vi "功率电压图.vi"(11 "功率控制表":refnum<vi>) -> ()   [LabVIEW 2015]
panel:
  out "XY图":cluster{i32[], dbl[]}[](graph)
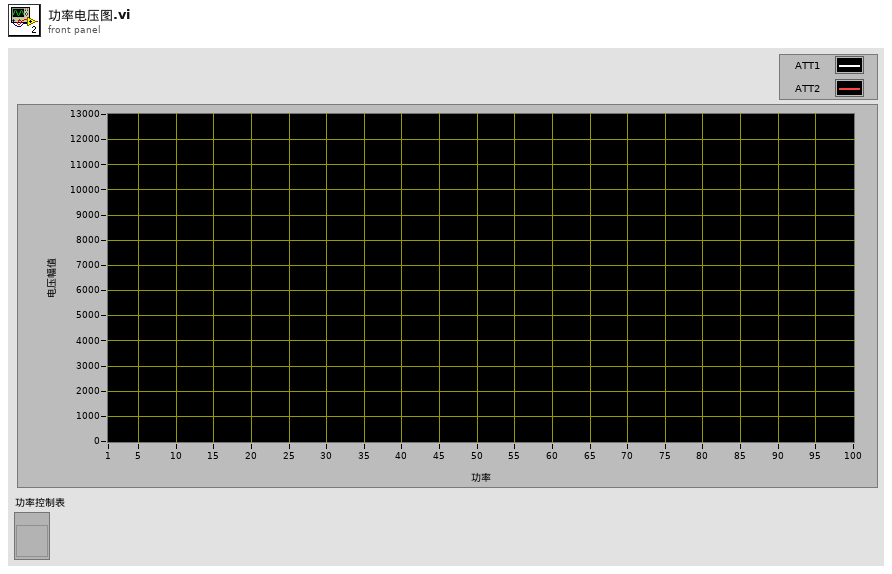
[diagram p1: front panel]
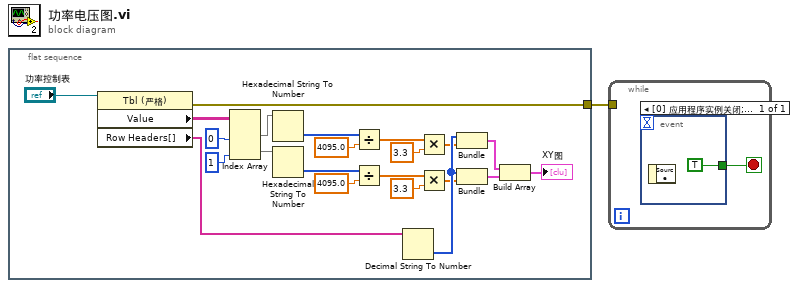
[diagram p0: block diagram]
diagram:
  n1 = flat-sequence {
    tunnel: [w12] -> w1
    frame #0 {
      n2 = property class="Tbl (严格)"(reference="功率控制表") -> (error out=w12:errorcluster, "Value"=w20:string[][], "Row Headers[]"=w21:string[])  [unwired: 1 in, 1 out]
      n3 = Index Array(array=w20, index (col) #1=0 ("禁用的索引 (列)"), index (col) #2=1 ("禁用的索引 (列)")) -> (element #1=w17:string[], element #2=w16:string[])  [unwired: 2 in]
      n4 = Hexadecimal String To Number(string=w17) -> (number=w8:u32[])  [unwired: 2 in, 1 out]
      n5 = Hexadecimal String To Number(string=w16) -> (number=w3:u32[])  [unwired: 2 in, 1 out]
      n6 = Divide(x=w8, y=4095.0) -> (x/y=w10:dbl[])
      n7 = Divide(x=w3, y=4095.0) -> (x/y=w5:dbl[])
      n8 = Decimal String To Number(string=w21) -> (number=w15:i32[])  [unwired: 2 in, 1 out]
      n9 = Multiply(x=w10, y=3.3) -> (x*y=w7:dbl[])
      n10 = Multiply(x=w5, y=3.3) -> (x*y=w2:dbl[])
      n11 = Bundle(w15, w7) -> (w23:cluster{i32[], dbl[]})  [unwired: 1 in]
      n12 = Bundle(w15, w2) -> (w14:cluster{i32[], dbl[]})  [unwired: 1 in]
      n13 = Build Array(w23, w14) -> (→"XY图":cluster{i32[], dbl[]}[])
    }
  }
  n14 = while {
    tunnel: w1 -> [_]
    stop <- w24 stop-if-true
    n15 = event shown="[0] 应用程序实例关闭;  前面板关闭" {
      selector: _ -> [_]
      dyn-events: _ -> [_]
      timeout: _ -> [_]
      tunnel: [TRUE] -> w24
      event Application Instance Close; Panel Close {
        n16 = event-data() -> ()  [unwired: 1 in, 1 out]
      }
    }
  }
